vi "setModulePath.vi"(8 "error in (no error)":errorcluster, 10 "modulePathStr":string, 11 "IInstanceBuilder in":refnum<class "IInstanceBuilder.lvclass">) -> (0 "error out":errorcluster, 3 "IInstanceBuilder out":refnum<class "IInstanceBuilder.lvclass">)   [LabVIEW 2022 SP3, in "openDAQ.lvlib" / "IBaseObject.lvlib" / "IInstanceBuilder.lvlib" / "IInstanceBuilder.lvclass"]
uses:
  <instrlib>/openDAQ/Public/Classes/IInstanceBuilder/IInstanceBuilder.lvclass
  C:/Program Files (x86)/National Instruments/LabVIEW 2022/instr.lib/openDAQ/Public/Classes/IBaseObject/IBaseObject.lvclass
  <instrlib>/openDAQ/Public/Classes/IBaseObject/IBaseObject.lvclass/IBaseObject.ctl
  <instrlib>/openDAQ/Public/Classes/IBaseObject/Accessor/Read reference.vi
  <instrlib>/openDAQ/Public/Classes/IBaseObject/Accessor/Write reference.vi
  <instrlib>/openDAQ/Public/Classes/daqCoreTypes/IString/IString.lvclass
  <instrlib>/openDAQ/Binaries/Windows/x86/copendaq32.dll
  <instrlib>/openDAQ/openDAQ.lvlib
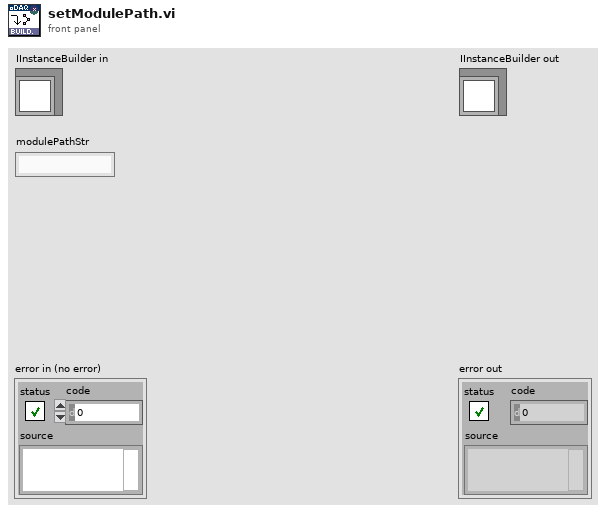
[diagram p1: front panel]
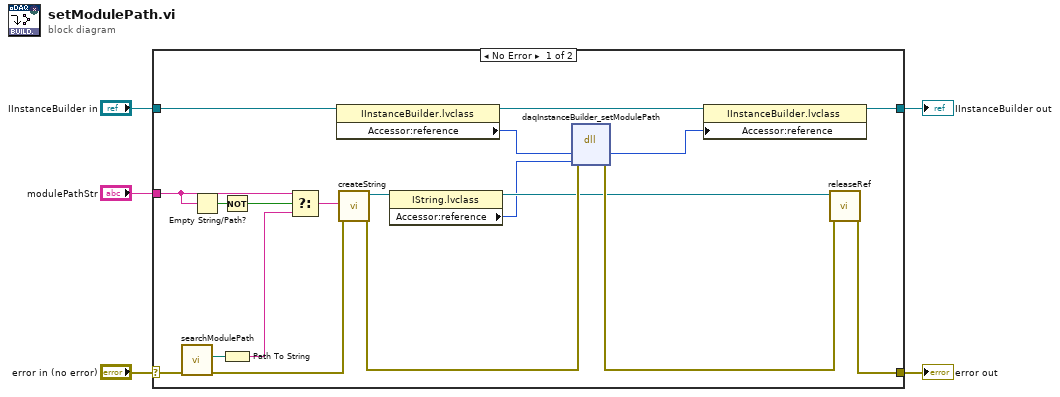
[diagram p0: block diagram]
diagram:
  n1 = case shown="No Error" "error in (no error)" {
    selector: "error in (no error)" -> [w13 w26]
    tunnel: [w14 w26] -> w4
    tunnel: [w18 w25] -> w2
    tunnel: "IInstanceBuilder in" -> [w19 w25]
    tunnel: "modulePathStr" -> [w7 _]
    frame No Error {
      n2 = call <instrlib>:"searchModulePath.vi"("error in (no error)"=w13) -> ("error out"=w12:errorcluster, "module path out"=w10:path)  [unwired: 9 in]
      n3 = Empty String/Path?(string/path=w7) -> (empty?=w11:bool)
      n4 = Not(x=w11) -> (.not. x?=w9:bool)
      n5 = Path To String(path=w10) -> (string=w8:string)
      n6 = Select(t=w7, s=w9, f=w8) -> (s? t:f=w6:string)
      n7 = property class="IInstanceBuilder.lvclass"(reference=w19) -> (reference out=w17:refnum<class "IInstanceBuilder.lvclass">, "Accessor:reference"=w16:i64)  [unwired: 1 in, 1 out]
      n8 = call <instrlib>:"createString.vi"("error in (no error)"=w12, "String"=w6) -> ("error out"=w23:errorcluster, "IString out"=w22:refnum<class "IString.lvclass">)  [unwired: 8 in]
      n9 = property class="IString.lvclass"(reference=w22) -> (reference out=w21:refnum<class "IString.lvclass">, "Accessor:reference"=w20:i64)  [unwired: 1 in, 1 out]
      n10 = dll-call lib="C:/Program Files (x86)/National Instruments/LabVIEW 2022/instr.lib/openDAQ/Binaries/Windows/x86/copendaq*.*" fn="daqInstanceBuilder_setModulePath"(error in=w23, "instanceBuilder"=w16, "modulePath"=w20) -> (error out=w24:errorcluster, "instanceBuilder"=w15:i64)  [unwired: 4 in, 1 out]
      n11 = property class="IInstanceBuilder.lvclass"(reference=w17, "Accessor:reference"=w15) -> (reference out=w18:refnum<class "IInstanceBuilder.lvclass">)  [unwired: 1 in, 1 out]
      n12 = call-dynamic "releaseRef.vi"("error in (no error)"=w24, "IBaseObject in"=w21) -> ("error out"=w14:errorcluster)  [unwired: 9 in]
    }
    frame Error {
    }
  }
  "error out" <- w4
  "IInstanceBuilder out" <- w2
